vi "Pack Data.vi"(8 "error in (no error)":errorcluster, 10 "packed data size (bits)":i32, 11 "unpacked data in":i16[](array[numeric])) -> (0 "error out":errorcluster, 3 "packed data out":i16[](array[numeric]))   [LabVIEW 2021, in "Digitizer Control.lvclass"]
doc: "Bit packs an array of integers into an array of 16-bit integers.\n\nInputs:\n\n<B>unpacked data in</B>: Array of integers containing the data to pack. The elements of the array are read LSB first.\n\n<B>packed data size (bits)</B>: The number of bits to keep from each <B>unpacked data in</B> array element.\n\nOutputs:\n\n<B>packed data out</B>: Array of I16s containing the packed data. The elements of the array are written LSB first."
uses:
  Digitizer Control.lvclass
  <vilib>/Utility/error.llb/Error Cluster From Error Code.vi
  <vilib>/ErrorRing/Error Ring.xnode
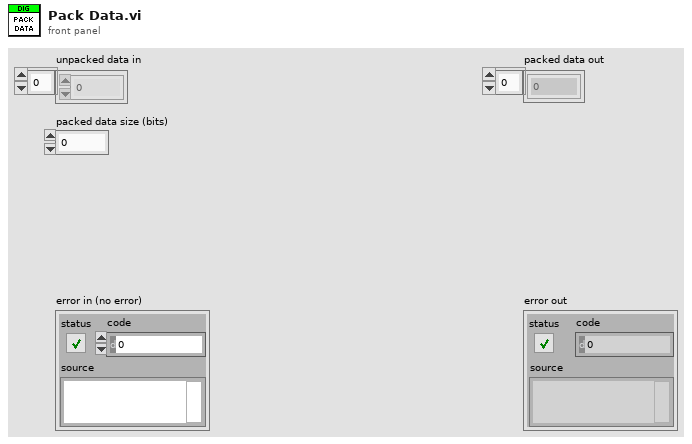
[diagram p1: front panel]
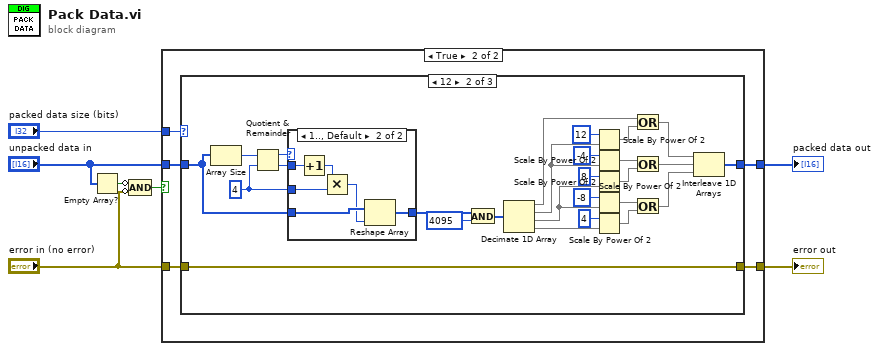
[diagram p0: block diagram]
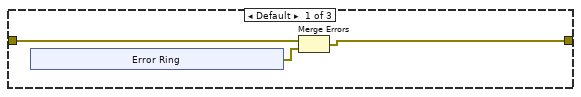
[diagram p3: hidden frame]
diagram:
  n1 = Empty Array?(array="unpacked data in") -> (empty?=w3:bool)
  n2 = Compound Arithmetic op=AND(invert w3, invert "error in (no error)") -> (w1:bool)
  n3 = case shown="True" w1 {
    tunnel: [w8 w13] -> w7
    tunnel: [_ w12] -> w6
    tunnel: "unpacked data in" -> [_ w10]
    tunnel: "packed data size (bits)" -> [_ w9]
    tunnel: "error in (no error)" -> [w8 w11]
    frame False {
    }
    frame True {
      n4 = case shown="12" w9 {
        tunnel: w11 -> [w16 w48 w57]
        tunnel: w10 -> [_ w29 w56]
        tunnel: [w14 w48 w57] -> w13
        tunnel: [_ w24 w56] -> w12
        frame Default {
          n5 = xnode "Error Ring"() -> ("error out"=w15:errorcluster)
          n6 = Merge Errors(w16, w15) -> (w14:errorcluster)
        }
        frame 12 {
          w26 = 4 ("y")
          n7 = Array Size(array=w29) -> (size(s)=w47:i32)
          n8 = Quotient & Remainder(x=w47, y=w26) -> (x-y*floor(x/y)=w27:i32, floor(x/y)=w28:i32)
          n9 = case shown="1.., Default" w27 {
            tunnel: w29 -> [w49 w54]
            tunnel: w28 -> [_ w55]
            tunnel: [w49 w50] -> w25
            tunnel: w26 -> [_ w52]
            frame 0 {
            }
            frame 1.., Default {
              n10 = Increment(x=w55) -> (x+1=w53:i32)
              n11 = Multiply(x=w53, y=w52) -> (x*y=w51:i32)
              n12 = Reshape Array(w54, w51) -> (w50:i16[])
            }
          }
          n13 = And(x=w25, y=i16 4095) -> (x .and. y?=w35:i16[])
          n14 = Decimate 1D Array(w35) -> (w34:i16[], w33:i16[], w23:i16[], w22:i16[])
          n15 = Scale By Power Of 2(n=i16 12 ("y"), x=w33) -> (x*2^n=w40:i16[])
          n16 = Scale By Power Of 2(n=i16 -4 ("y"), x=w33) -> (x*2^n=w39:i16[])
          n17 = Scale By Power Of 2(n=i16 8 ("y"), x=w23) -> (x*2^n=w38:i16[])
          n18 = Scale By Power Of 2(n=i16 -8 ("y"), x=w23) -> (x*2^n=w37:i16[])
          n19 = Scale By Power Of 2(n=i16 4 ("y"), x=w22) -> (x*2^n=w36:i16[])
          n20 = Or(x=w34, y=w40) -> (x .or. y?=w32:i16[])
          n21 = Or(x=w39, y=w38) -> (x .or. y?=w31:i16[])
          n22 = Or(x=w37, y=w36) -> (x .or. y?=w30:i16[])
          n23 = Interleave 1D Arrays(w32, w31, w30) -> (w24:i16[])
        }
        frame 16 {
        }
      }
    }
  }
  "error out" <- w7
  "packed data out" <- w6
